vi "DUC (Single Channel).vi"(0 "data in":T4, 1 "reset":bool, 5 "enabled":bool, 9 "input valid":bool, 11 "DUC Parameters":T1={"frequency shift"=0.0, "impairments"={"inline gain I"=0.9999923706054688, "inline gain Q"=0.9999923706054688, "cross gain I"=0.0, "cross gain Q"=0.0, "pre-gain offset I"=0.0, "pre-gain offset Q"=0.0, "post-gain offset I"=0.0, "post-gain offset Q"=0.0}, "phase"=0.0, "input sample rate"=0.0, "gain"={"gain I"=1.0, "gain Q"=1.0}, "delay"=0.0} {"frequency shift" format="%#.48g"}) -> (4 "I data out":i16, 6 "Q data out":i16, 10 "output valid":bool, 13 "dsp reset done":bool, 14 "ready for input":bool, 15 "number of overflows":u64)   [LabVIEW 2023]
doc: "Digital upconverter (DUC) for a single channel. Implemented with FPGA-based DSP."
uses:
  <instrlib>/_niInstr/Basic Elements/v1/FPGA/Private/Count Up U64.vi
  <instrlib>/_niInstr/DSP/v1/FPGA/Public/Sub VIs/Fractional Interpolator/Fractional Interpolator - 1 spc - 2x oc.vi
  <instrlib>/_niInstr/DSP/v1/FPGA/Public/Sub VIs/Digital Gain/Digital Gain - 1 spc.vi
  <instrlib>/_niInstr/DSP/v1/FPGA/Public/Sub VIs/Frequency Shift/Frequency Shift - 1 spc.vi
  <instrlib>/_niInstr/DSP/v1/FPGA/Public/Sub VIs/IQ Impairments/IQ Impairments - 1 spc.vi
  <instrlib>/_niInstr/DSP/v1/Shared/Public/IQ Data.ctl
  <instrlib>/_niInstr/DSP/v1/FPGA/Public/Sub VIs/Data Conversion/IQ to I16 - 1 spc - S18.1.vi
  <instrlib>/_niInstr/DSP/v1/Shared/Public/IQ Impairments.ctl
  <instrlib>/_niInstr/DSP/v1/Shared/Public/IQ Gain.ctl
  <instrlib>/niUSRP/Reference FPGA/USRPRIO Sample VIs/FPGA/SubVIs/DUC Parameters.ctl
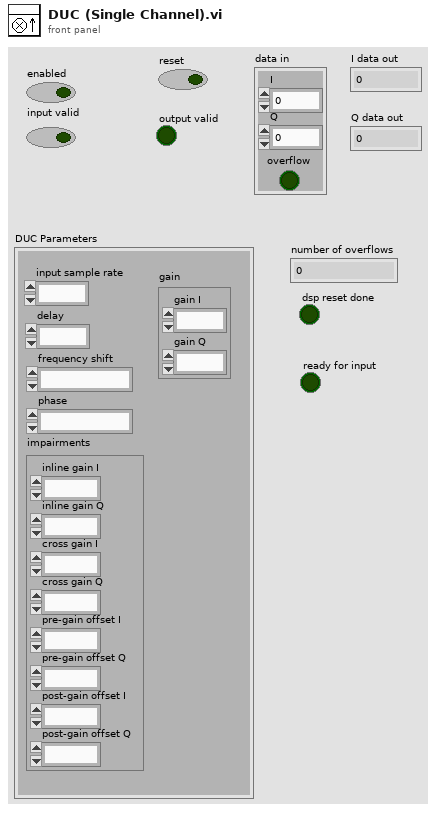
[diagram p1: front panel]
types:
  T1 = typedef "DUC Parameters.ctl" = cluster{"frequency shift":fxp<+/-,48,0>, "impairments":T2, "phase":fxp<+/-,21,0>, "input sample rate":fxp<+,48,1>, "gain":T3, "delay":fxp<+/-,18,0>}
  T2 = typedef "niInstr DSP v1 Shared.lvlib/IQ Impairments.ctl" = cluster{"inline gain I":fxp<+/-,18,1>, "inline gain Q":fxp<+/-,18,1>, "cross gain I":fxp<+/-,18,1>, "cross gain Q":fxp<+/-,18,1>, "pre-gain offset I":fxp<+/-,18,1>, "pre-gain offset Q":fxp<+/-,18,1>, "post-gain offset I":fxp<+/-,18,1>, "post-gain offset Q":fxp<+/-,18,1>}
  T3 = typedef "niInstr DSP v1 Shared.lvlib/IQ Gain.ctl" = cluster{"gain I":fxp<+/-,24,3>, "gain Q":fxp<+/-,24,3>}
  T4 = typedef "niInstr DSP v1 Shared.lvlib/IQ Data.ctl" = cluster{"I":fxp<+/-,18,1>, "Q":fxp<+/-,18,1>, "overflow":bool}
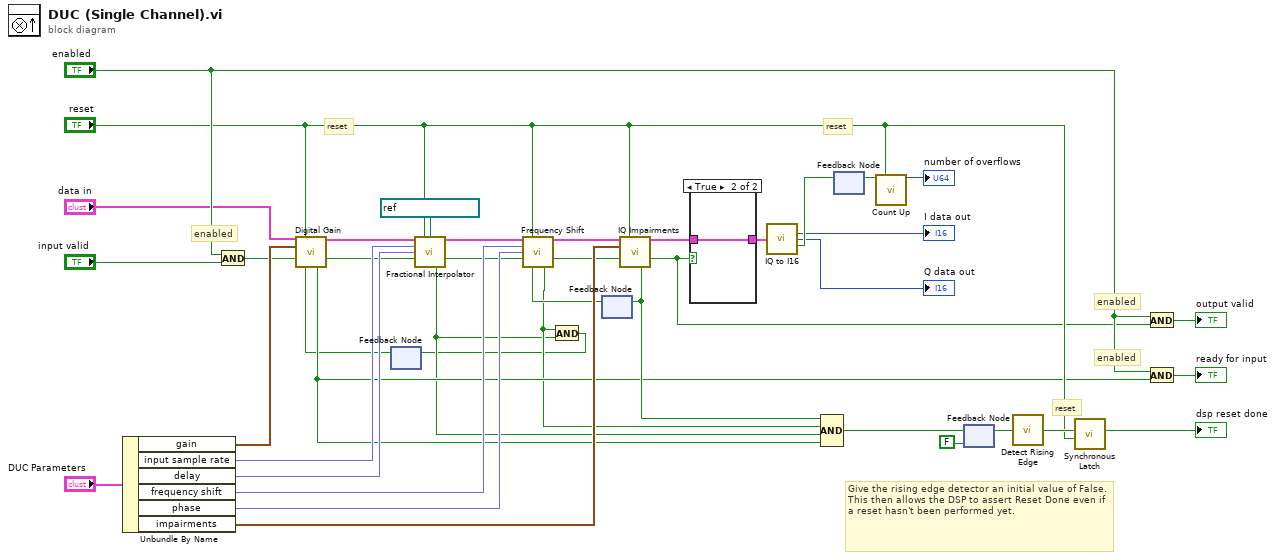
[diagram p0: block diagram]
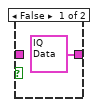
[diagram p2: hidden frame]
diagram:
  # "Give the rising edge detector an initial value of False.  This then allows the DSP to assert Reset Done even if a reset hasn't been performed yet."
  # "enabled"
  # "reset"
  # "reset"
  # "reset"
  # "enabled"
  # "enabled"
  n1 = Unbundle By Name("DUC Parameters") -> ("gain"=w33:T3, "input sample rate"=w27:fxp<+,48,1>, "delay"=w26:fxp<+/-,18,0>, "frequency shift"=w25:fxp<+/-,48,0>, "phase"=w24:fxp<+/-,21,0>, "impairments"=w23:T2)
  n2 = And(x="enabled", y="input valid") -> (x .and. y?=w22:bool)
  n3 = feedback #1() -> (w1:bool)  [unwired: 1 in]
  n4 = call-poly <instrlib>:"Digital Gain.vi"("data in"="data in", "reset"="reset", "gain"=w33, "input valid"=w22, "ready for output (T)"=w1) -> ("data out"=w14:T4, "output valid"=w13:bool, "ready for input"=w6:bool)  [unwired: 8 in]
  n5 = call-poly <instrlib>:"Fractional Interpolator.vi"("data in"=w14, "reset"="reset", "clock x 2"=refnum<k21> "Data Clock x2" ("oversample clock"), "input sample rate"=w27, "delay"=w26, "input valid"=w13) -> ("data out"=w18:T4, "output valid"=w17:bool, "ready for input"=w3:bool)  [unwired: 6 in, 1 out]
  n6 = feedback #2() -> (w11:bool)  [unwired: 1 in]
  n7 = call-poly <instrlib>:"Frequency Shift.vi"("data in"=w18, "reset"="reset", "frequency shift"=w25, "phase"=w24, "input valid"=w17, "ready for output (T)"=w11) -> ("data out"=w16:T4, "output valid"=w15:bool, "ready for input"=w4:bool)  [unwired: 7 in]
  n8 = And(x=w4, y=w3) -> (x .and. y?=w2:bool)
  n9 = feedback-in #1(w2) -> ()
  n10 = call-poly <instrlib>:"IQ Impairments.vi"("data in"=w16, "reset"="reset", "impairments"=w23, "input valid"=w15) -> ("data out"=w20:T4, "output valid"=w21:bool, "ready for input"=w7:bool)  [unwired: 9 in]
  n11 = feedback-in #2(w7) -> ()
  n12 = case shown="True" w21 {
    tunnel: w20 -> [_ w43]
    tunnel: [T4 {"I"=0.0, "Q"=0.0, "overflow"=FALSE} ("data out") w43] -> w19
    frame False {
    }
    frame True {
    }
  }
  n13 = call-poly <instrlib>:"IQ to I16.vi"("IQ"=w19) -> ("I"=→"I data out":i16, "Q"=→"Q data out":i16, "overflow"=w30:bool)  [unwired: 12 in]
  n14 = Compound Arithmetic op=AND(w7, w4, w3, w6) -> (w5:bool)
  n15 = feedback #3() -> (w37:bool)  [unwired: 1 in]
  n16 = feedback-in #3(w30) -> ()
  n17 = call-poly <instrlib>:"Count Up.vi"("increment"=w37, "reset"="reset") -> ("count out"=→"number of overflows":u64)  [unwired: 13 in]
  n18 = feedback-in #4(w5) -> ()
  n19 = feedback #4(FALSE ("ready for input")) -> (w9:bool)
  n20 = call <instrlib>:"Detect Rising Edge.vi"("signal"=w9) -> ("edge detected"=w40:bool)  [unwired: 14 in]
  n21 = call <instrlib>:"Synchronous Latch.vi"("clear"="reset", "set"=w40) -> ("out"=→"dsp reset done":bool)  [unwired: 9 in]
  n22 = And(x="enabled", y=w21) -> (x .and. y?=→"output valid":bool)
  n23 = And(x="enabled", y=w6) -> (x .and. y?=→"ready for input":bool)
